vi "1D Kalman - Update Measurement Noise.vi"(10 "Measurement Noise (non-correlated)":dbl[](array[numeric]), 11 "Second-Order Statistics Noise Model In":T1 {"N" format="%#.2g"; "R" format="%#.2g"; "E{v}" format="%#.2g"; "E{w}" format="%#.2g"; "Q" format="%#.2g"}) -> (3 "Second-Order Statistics Noise Model out":T1 {"N" format="%#.2g"; "R" format="%#.2g"; "E{v}" format="%#.2g"; "E{w}" format="%#.2g"; "Q" format="%#.2g"})   [LabVIEW 2017]
uses:
  <vilib>/addons/Control Design/_Stochastic Systems/Stochastic Systems.llb/Stochastic Systems SubVIs/cd_Second-Order Statistics Noise Model.ctl
  <vilib>/addons/Control Design/_Stochastic Systems/NI_CD_Stochastic Systems.lvlib
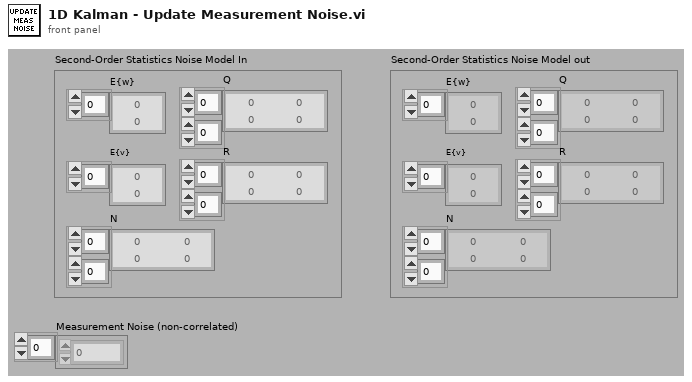
[diagram p1: front panel]
types:
  T1 = typedef "NI_CD_Stochastic Systems.lvlib/cd_Second-Order Statistics Noise Model.ctl" = cluster{"Q":dbl[][], "E{w}":dbl[], "E{v}":dbl[], "R":dbl[][], "N":dbl[][]}
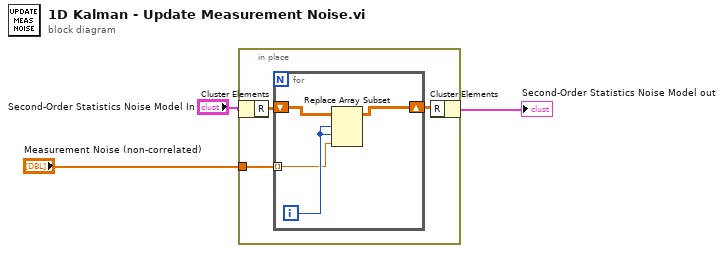
[diagram p0: block diagram]
diagram:
  n1 = in-place {
    in-place-border: "Measurement Noise (non-correlated)" -> [w6]
    n2 = in-place-cluster #1("Second-Order Statistics Noise Model In") -> ("R"=w5:dbl[][])
    n3 = for {
      tunnel: w6 -> [w8] mode=indexing
      shift-right: [w7] -> w4
      shift-left: w5 -> [w10]
      i -> [w9]
      n4 = Replace Array Subset(array=w10, new element=w8, index (row)=w9, index (col)=w9) -> (w7:dbl[][])
    }
    n5 = in-place-cluster #1("R"=w4) -> (→"Second-Order Statistics Noise Model out":T1)
  }
